vi "uintAdd.vi"(8 "Error in (no error)":errorcluster, 10 "Uint2 in":refnum<class "UintClass.lvclass">, 11 "Uint1 in":refnum<class "UintClass.lvclass">) -> (0 "Error out":errorcluster, 1 "Timing":u32, 3 "Uint1 + Uint2":refnum<class "UintClass.lvclass">)   [LabVIEW 2011, in "UintClass.lvclass"]
uses:
  UintClass.lvclass
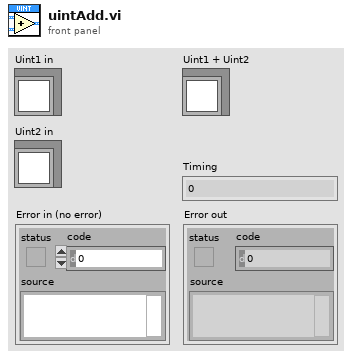
[diagram p1: front panel]
types:
  T1 = typedef "UintClass.lvclass/enumBase.ctl" = u16
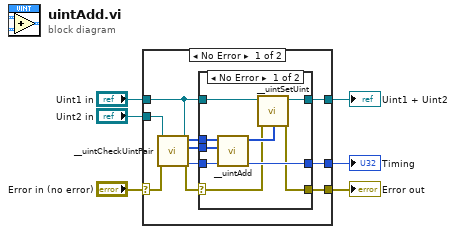
[diagram p0: block diagram]
diagram:
  n1 = case shown="No Error" "Error in (no error)" {
    selector: "Error in (no error)" -> [w13 w27]
    tunnel: [w11 w27] -> w5
    tunnel: "Uint2 in" -> [w14 _]
    tunnel: "Uint1 in" -> [w7 _]
    tunnel: [w16 _] -> w2
    tunnel: [w15 _] -> w1
    frame No Error {
      n2 = call "__uintCheckUintPair.vi"("Error in (no error)"=w13, "Uint2 in"=w14, "Uint1 in"=w7) -> ("Error out"=w12:errorcluster, "Uint2 out"=w9:u8[], "Uint1 out"=w10:u8[], "Base out"=w8:T1)  [unwired: 5 in]
      n3 = case shown="No Error" w12 {
        selector: w12 -> [w18 w26]
        tunnel: [w25 _] -> w16
        tunnel: [w23 _] -> w15
        tunnel: [w17 w26] -> w11
        tunnel: w10 -> [w22 _]
        tunnel: w9 -> [w21 _]
        tunnel: w8 -> [w20 _]
        tunnel: w7 -> [w19 _]
        frame No Error {
          n4 = call "__uintAdd.vi"("Base (decimal)"=w20, "Uint2 in"=w21, "Uint1 in"=w22) -> ("Timing"=w25:u32, "Uint1 + Uint2"=w24:u8[])  [unwired: 7 in]
          n5 = call "__uintSetUint.vi"("Error in (no error)"=w18, 10:"Uint in"=w24, 11:"Uint in"=w19) -> ("Error out"=w17:errorcluster, "Uint out"=w23:refnum<class "UintClass.lvclass">)  [unwired: 7 in]
        }
        frame Error {
        }
      }
    }
    frame Error {
    }
  }
  "Error out" <- w5
  "Uint1 + Uint2" <- w1
  "Timing" <- w2
